vi "Set Device Information.vi"() -> (0 "error out":errorcluster, 2 "Workspace Info":T1={"Device Name"="test", "Device Info"="test", "Path"=path "C:/Users/gio/Desktop/test"}, 3 "OK?":bool)   [LabVIEW 2014]
uses:
  Save Data/SaveData Workspace Info.ctl
  <vilib>/Utility/sysdir.llb/System Directory Type.ctl
panel:
  in  "Device ID":string
  in  "Cancel":bool
  out "Path":path
  in  "OK Button":bool
  in  "Device Information":string
  # "LICENSED MATERIALS – PROPERTY OF IBM\nCopyright IBM Corp. 2016,\nALL RIGHTS RESERVED"
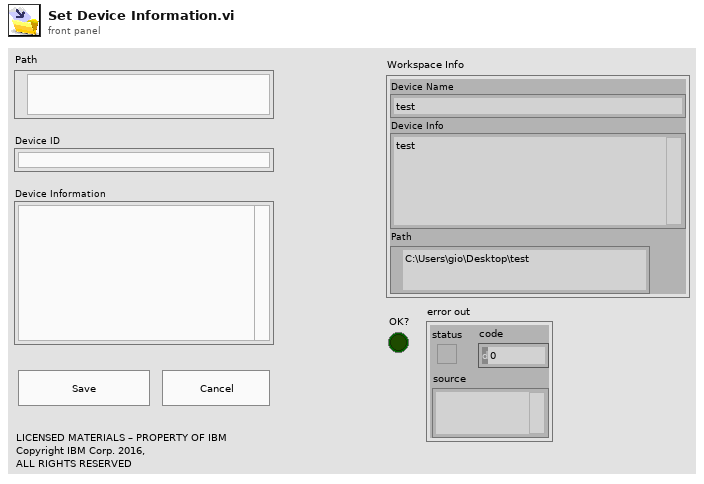
[diagram p1: front panel]
types:
  T1 = typedef "SaveData Workspace Info.ctl" = cluster{"Device Name":string, "Device Info":string, "Path":path}
  T2 = typedef "System Directory Type.ctl" = i32
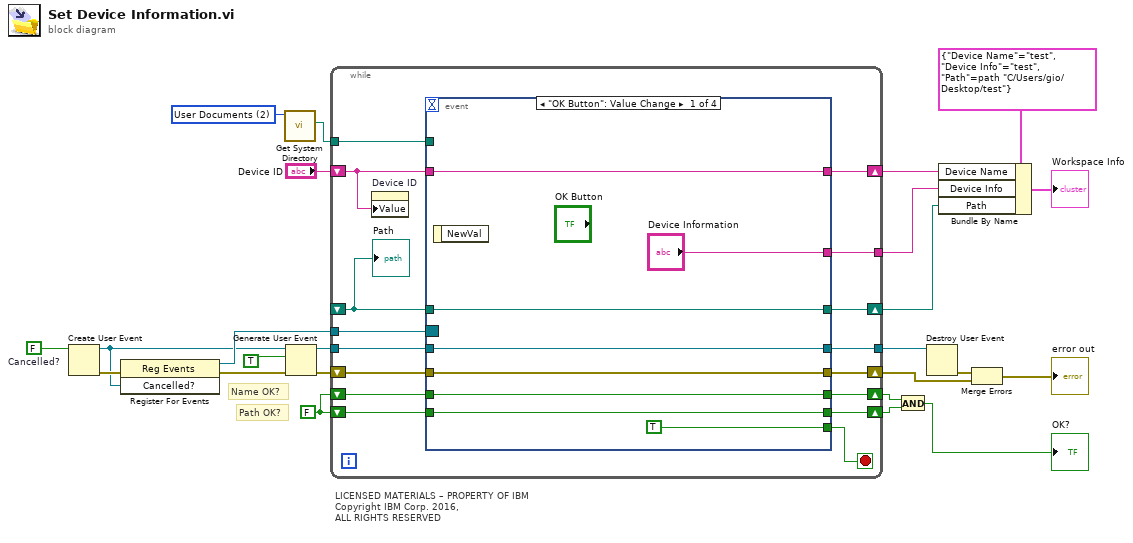
[diagram p0: block diagram]
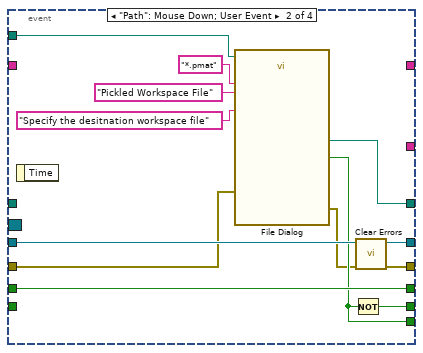
[diagram p2: hidden frame]
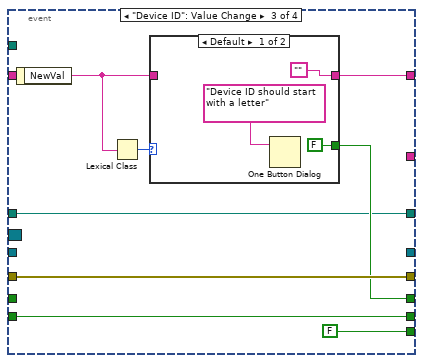
[diagram p3: hidden frame]
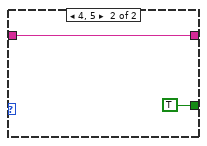
[diagram p4: hidden frame]
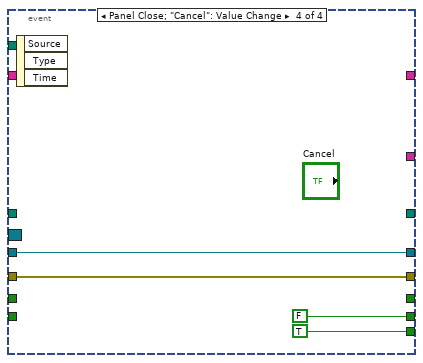
[diagram p5: hidden frame]
diagram:
  w2 = T2 2 items=["User Home"=0, "User Desktop"=1, "User Documents"=2, "User Application Data"=3, "User Preferences"=4, "User Temporary"=5, "Public Documents"=6, "Public Application Data"=7, "Public Preferences"=8, "Public Cache"=13, "System Core Libraries"=9, "System Installed Libraries"=10, "Application Files"=11, "Boot Volume Root"=12] ("system directory type")
  w7 = FALSE ("event data")
  w21 = FALSE  # Cancelled?
  # "LICENSED MATERIALS – PROPERTY OF IBM\nCopyright IBM Corp. 2016,\nALL RIGHTS RESERVED"
  # "Name OK?"
  # "Path OK?"
  n1 = Create User Event(user event datatype=w21) -> (user event=w13:refnum<user-event>, error out=w20:errorcluster)  [unwired: 1 in]
  n2 = register-events(error in=w20, w13) -> (reference out=w19:refnum<event-registration>, error out=w12:errorcluster)  [unwired: 1 in]
  n3 = call <vilib>:"Get System Directory.vi"("system directory type"=w2) -> ("system directory"=w1:path)  [unwired: 10 in]
  n4 = Generate User Event(user event=w13, event data cluster=TRUE ("event data"), error in=w12) -> (user event out=w10:refnum<user-event>, error out=w11:errorcluster)  [unwired: 1 in]
  n5 = while {
    shift-right: [w33] -> w22
    shift-left: _ -> [w39]
    tunnel: w19 -> [w37]
    shift-right: [w32] -> w16
    shift-left: w11 -> [w36]
    tunnel: w10 -> [w35]
    tunnel: [w34] -> w18
    tunnel: [w30] -> w8
    tunnel: w1 -> [w29]
    shift-right: [w31] -> w9
    shift-left: "Device ID" -> [w25]
    shift-right: [w38] -> w3
    shift-left: w7 -> [w28]
    shift-right: [w26] -> w4
    shift-left: w7 -> [w27]
    stop <- w40 stop-if-true
    n6 = property on="Device ID" class="Str"("Value"=w25) -> ()  [unwired: 2 in, 2 out]
    n7 = event shown="[0] \"OK Button\": Value Change" {
      selector: w37 -> [_ _ _ _]
      dyn-events: _ -> [_ _ _ _]
      timeout: _ -> [_ _ _ _]
      tunnel: [TRUE w52 FALSE ("event data") TRUE] -> w40
      tunnel: [w48 w57 w61 _] -> w33
      tunnel: w39 -> [w48 _ w61 _]
      tunnel: [w41 w53 w62 FALSE] -> w38
      tunnel: w36 -> [w46 w51 w65 w75]
      tunnel: [w46 w49 w65 w75] -> w32
      tunnel: w35 -> [w45 w55 _ w74]
      tunnel: [w45 w55 _ w74] -> w34
      tunnel: [w43 _ w67 _] -> w31
      tunnel: ["Device Information" _ _ _] -> w30
      tunnel: w29 -> [_ w56 _ _]
      tunnel: w25 -> [w43 _ _ _]
      tunnel: w28 -> [w41 _ w62 _]
      tunnel: w27 -> [w42 w54 _ _]
      tunnel: [w42 w54 w63 _] -> w26
      event "OK Button": Value Change {
        n8 = event-data() -> ()  [unwired: 2 out]
      }
      event "Path": Mouse Down; User Event {
        n9 = event-data() -> ()  [unwired: 2 out]
        n10 = call "File Dialog"("start path"=w56, "prompt"="Specify the desitnation workspace file", "error in"=w51, "pattern (all files)"="*.pmat", "pattern label"="Pickled Workspace File") -> ("selected path"=w57:path, "cancelled"=w52:bool, "error out"=w50:errorcluster)  [unwired: 2 in, 6 out]
        n11 = Not(x=w52) -> (.not. x?=w53:bool)
        n12 = call <vilib>:"Clear Errors.vi"("error in (no error)"=w50) -> ("error out"=w49:errorcluster)  [unwired: 5 in, 1 out]
      }
      event "Device ID": Value Change {
        n13 = event-data() -> ("NewVal"=w64:string)  [unwired: 1 out]
        n14 = Lexical Class(1:w64) -> (0:w68:i16)
        n15 = case shown="Default" w68 {
          tunnel: w64 -> [_ w73]
          tunnel: ["" w73] -> w67
          tunnel: [FALSE ("event data") TRUE ("event data")] -> w63
          frame Default {
            n16 = One Button Dialog(message="Device ID should start with a letter") -> ()  [unwired: 1 in, 1 out]
          }
          frame 4, 5 {
          }
        }
      }
      event Panel Close; "Cancel": Value Change {
        n17 = event-data() -> ()  [unwired: 4 out]
      }
    }
    "Path" <- w39
  }
  n18 = And(x=w4, y=w3) -> (x .and. y?=→"OK?":bool)
  n19 = Destroy User Event(user event=w18) -> (error out=w17:errorcluster)  [unwired: 1 in]
  n20 = Bundle By Name(cluster=T1 {"Device Name"="test", "Device Info"="test", "Path"=path "C:/Users/gio/Desktop/test"} ("Instrument Sequence - Workspace Info 2"), "Device Name"=w9, "Device Info"=w8, "Path"=w22) -> (→"Workspace Info":T1)
  n21 = Merge Errors(w17, w16) -> (→"error out":errorcluster)
